vi "Scan_change.vi"() -> ()   [LabVIEW 2022 SP3]
uses:
  <vilib>/userdefined/High Color/IMAQdx.ctl
  <vilib>/vision/driver/IMAQdx.llb/IMAQdx Acquisition Mode.ctl
  <vilib>/vision/driver/IMAQdx.llb/IMAQdx Buffer Number Mode.ctl
  <vilib>/Platform/TimedLoop/XDataNode/timing_clust.ctl
  <vilib>/Platform/TimedLoop/XDataNode/nitl_modes.ctl
  <vilib>/Platform/TimedLoop/XDataNode/wakeup.ctl
  <vilib>/Utility/file.llb/Write To Spreadsheet File (DBL).vi
  <vilib>/Utility/file.llb/Write To Spreadsheet File (I64).vi
  <vilib>/Platform/TimedLoop/XDataNode/XDataNode.xnode
  <vilib>/vision/driver/NI_Vision_Acquisition_Software.lvlib
  <resource>/objmgr/IMAQImage.rc
  <vilib>/Platform/TimedLoop/XDataNode/XDNodeRunTimeDep.lvlib
panel:
  in  "ExitSendCmd":bool
  out "Current File":path
  in  "Root File Name":string="Sample"
  in  "Display as wavelength?":bool=TRUE
  out "X axis":sgl[](array[numeric])
  in  "Tab Control":enum32{"Scan", "Motors"}(tab)
  in  "Release Scan":bool
  in  "Save Option":bool=TRUE
  out "Remaining Minutes":i32
  out "Progress Bar":dbl(slide) scale=0.0..1.0
  in  "Sample #":u16
  out "Cross Plane Length (mm)":sgl=128.0 format="%.3f"
  out "Scan Plane Length (mm)":sgl=128.0 format="%.3f"
  in  "Distance between\nscan lines (mm)":sgl=1.0 min=0.06 max=1000 step=0.06
  in  "Distance between\nplanes (mm)":sgl=1.0 min=0.06 max=1000 step=0.06
  in  "number of planes":u16=1660
  in  "lines per plane":u16=1660 min=1
  out "current plane":u16
  out "current line":u16
  in  "Abort":bool
  in  "start scan":bool
  out "Image":T1(plugin-control)
  out "Spectra":T2(graph)
  in  "Save Folder":path=path "C:/Scan Test"
  in  "Average#":i32=1 min=1
  in  "Exposure (*2.375 ms)":u16=2 format="%.3f"
  in  "Old way (T)/New Way (F)":bool=TRUE
  in  "Plane Axis":refnum<k7>(container)
  in  "Line axis":refnum<k7>(container)
  in  "Home Seq":bool
  in  "Go Home":bool
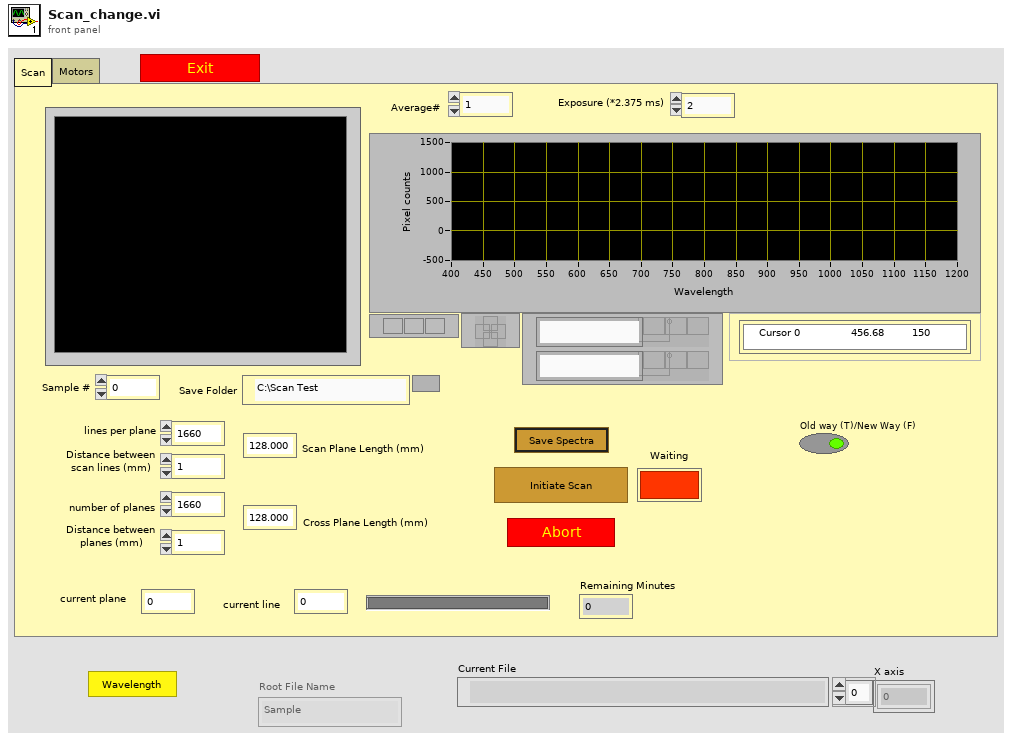
[diagram p1: front panel]
types:
  T1 = typedef "IMAQ Image.ctl" = refnum<image>
  T2 = cluster{"X axis":sgl[], "Spectral Amplitude":dbl[]}
  T3 = typedef "NI_Vision_Acquisition_Software.lvlib/IMAQdx Acquisition Mode.ctl" = enum32{"One Shot", "Continuous"}
  T4 = typedef "IMAQdx.ctl" = refnum<k21>
  T5 = typedef "NI_Vision_Acquisition_Software.lvlib/IMAQdx Buffer Number Mode.ctl" = enum32{"Next", "Last", "Buffer Number", "Every", "Last New"}
  T6 = enum16{"open", "replace", "create", "open or create", "replace or create", "replace or create with confirmation"}
  T7 = typedef "XDNodeRunTimeDep.lvlib/timing_clust.ctl" = cluster{"Expected End [f-1]":u64, "Actual End [f-1]":u64, "Finished Late? [f-1]":bool, "Expected End [i-1]":u64, "Actual End [i-1]":u64, "Finished Late? [i-1]":bool, "Expected Start [i]":u64, "Actual Start [i]":u64, "Expected Start [f]":u64, "Actual Start [f]":u64, "Source Name":string, "Structure Name":string, "Period":i64, "Deadline":i64, "Offset":i64, "Start":i64, "Priority":i32, "Timeout":i32, "Mode":T8, "Wakeup Reason":T9, "Error":errorcluster, "Source Type":string, "Secondary Source Type":string, "Global End Time":u64, "Global Start Time":u64, "Frame Duration":u64, "Iteration Duration":u64, "Assigned CPU":i32, "I/O Scan Engine Mode":u32}
  T8 = typedef "XDNodeRunTimeDep.lvlib/nitl_modes.ctl" = enum32{"No Change", "Process missed periods, maintain original phase", "Discard missed periods, maintain original phase", "Process missed periods, ignore original phase", "Discard missed periods, ignore original phase"}
  T9 = typedef "XDNodeRunTimeDep.lvlib/wakeup.ctl" = enum32{"Normal", "Aborted", "Asynchronous wakeup", "Timing source error", "Timed loop error", "Timeout"}
  T10 = enum16{"big-endian, network order", "native, host order", "little-endian"}
  T11 = typedef "Image Type" = u32
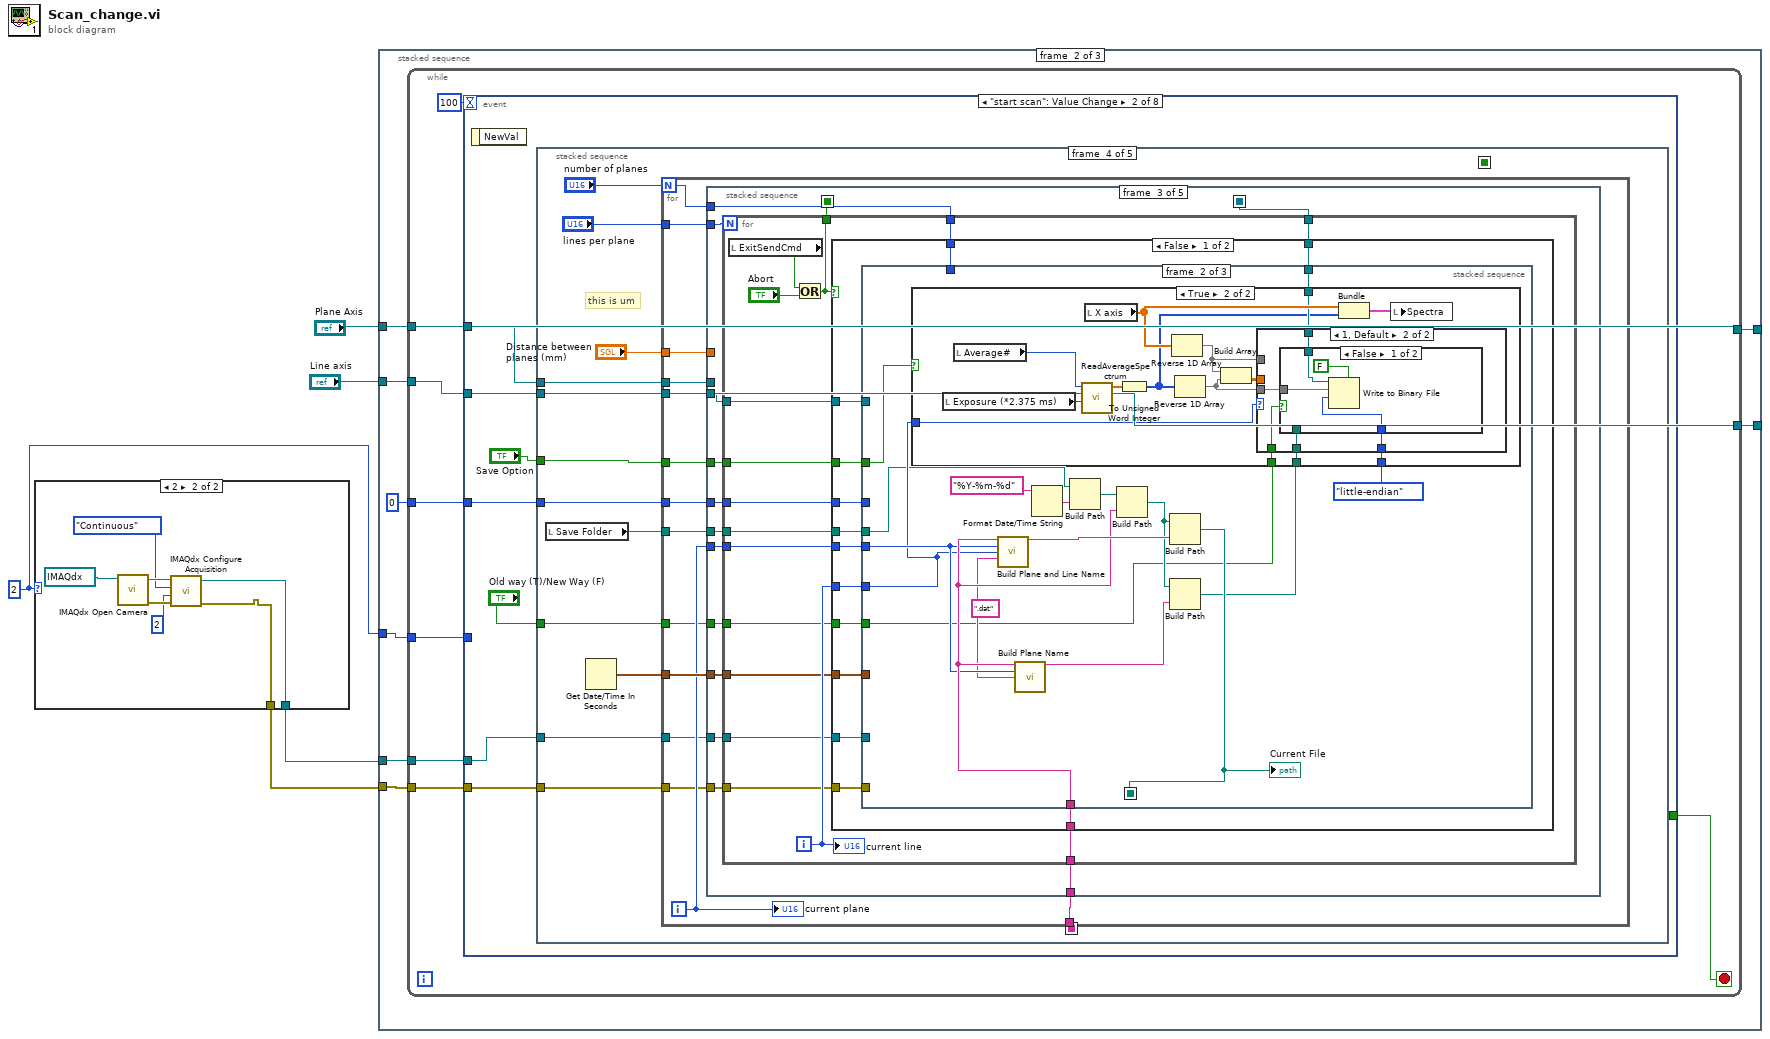
[diagram p0: block diagram]
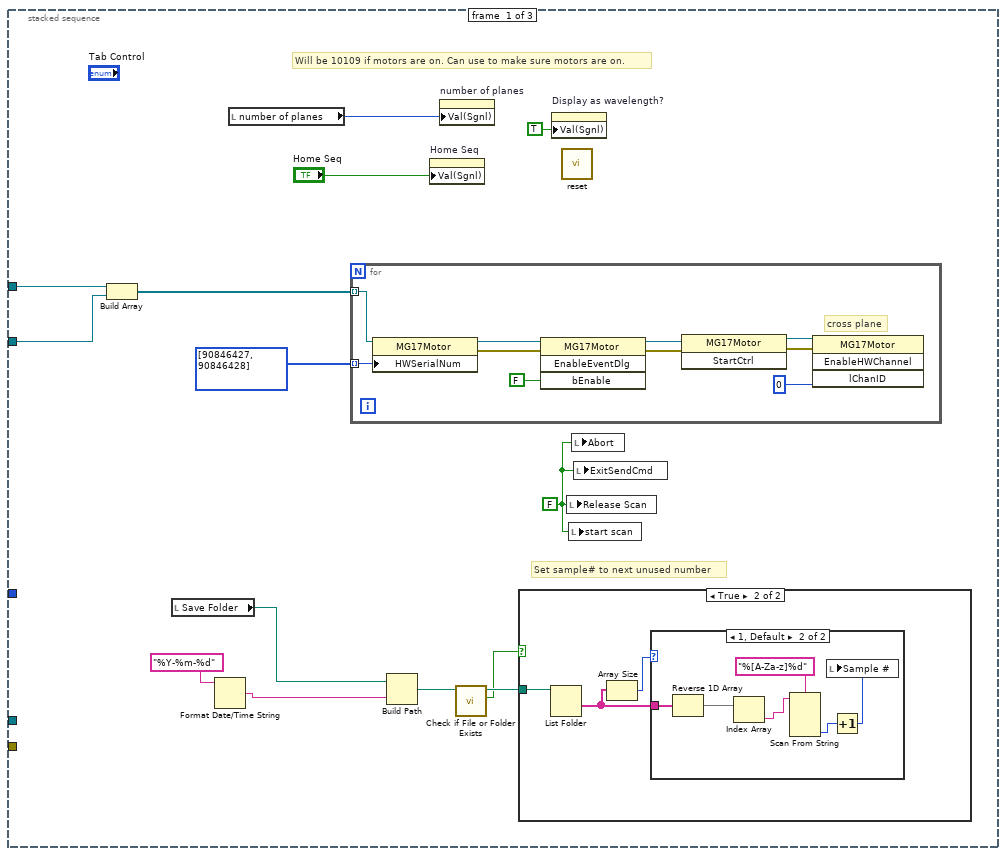
[diagram p3: hidden frame]
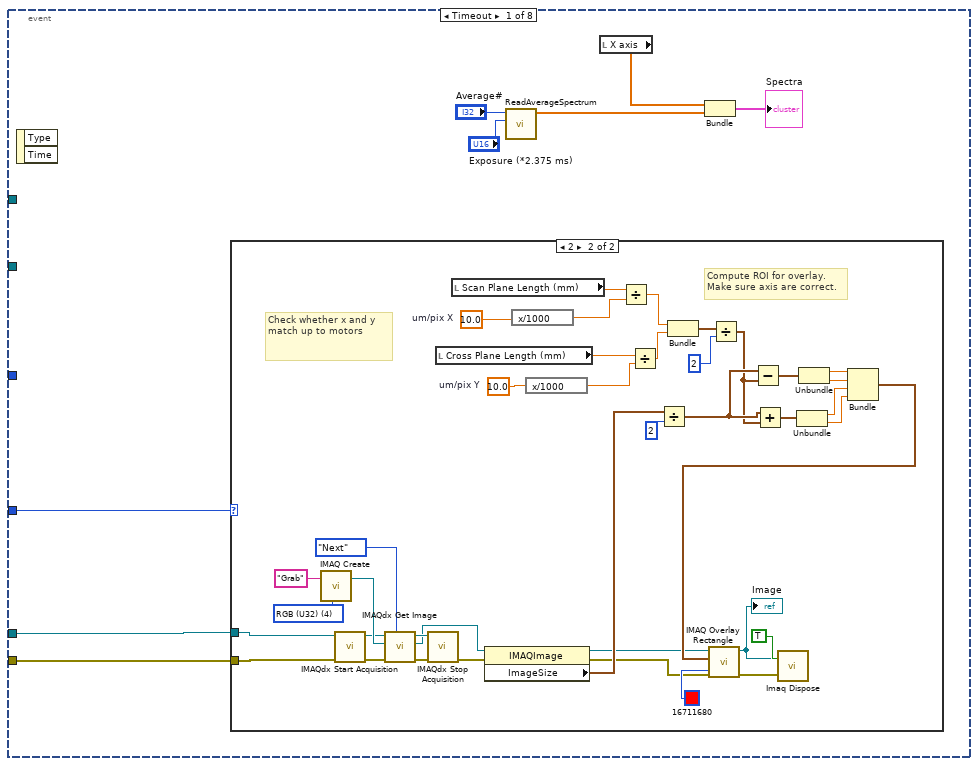
[diagram p6: hidden frame]
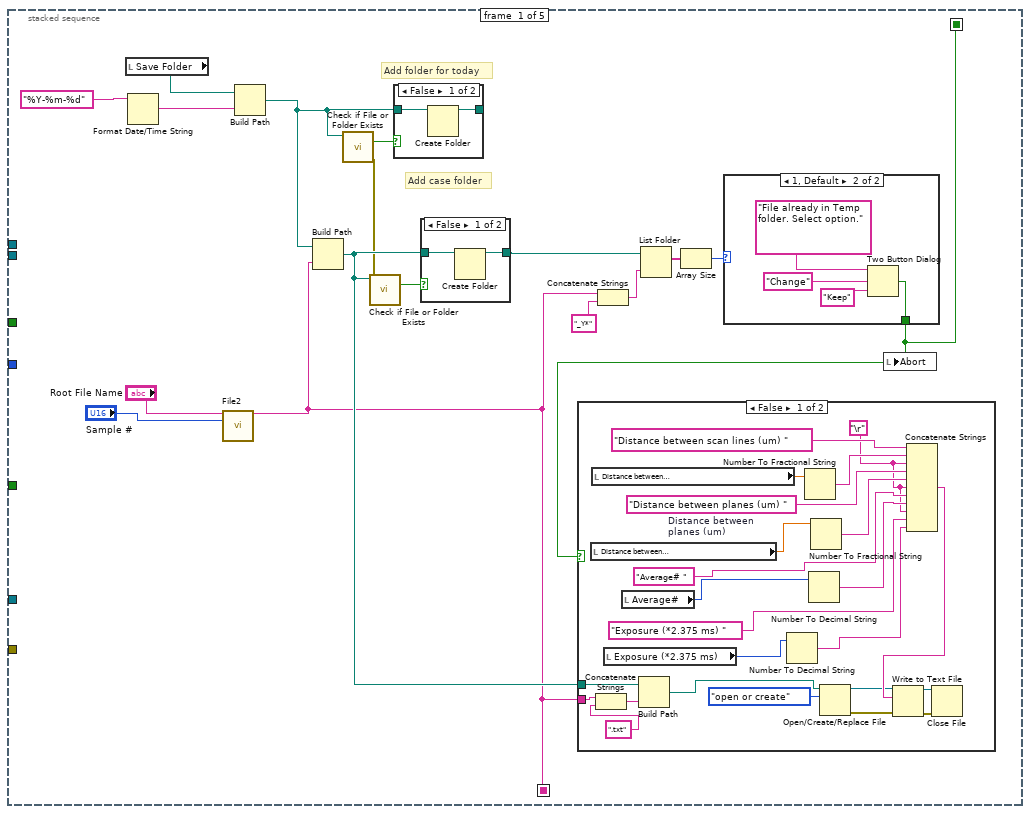
[diagram p8: hidden frame]
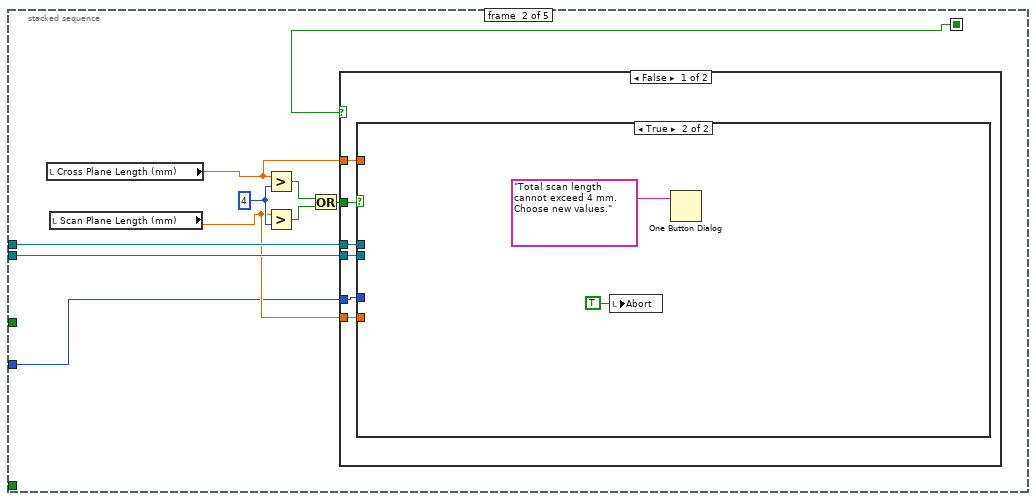
[diagram p13: hidden frame]
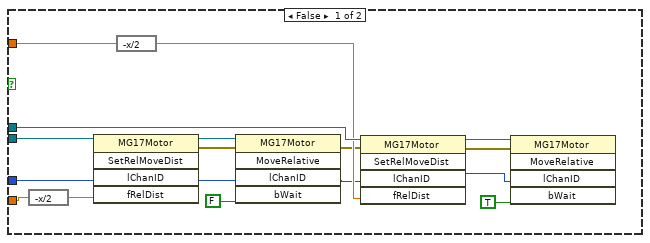
[diagram p14: hidden frame]
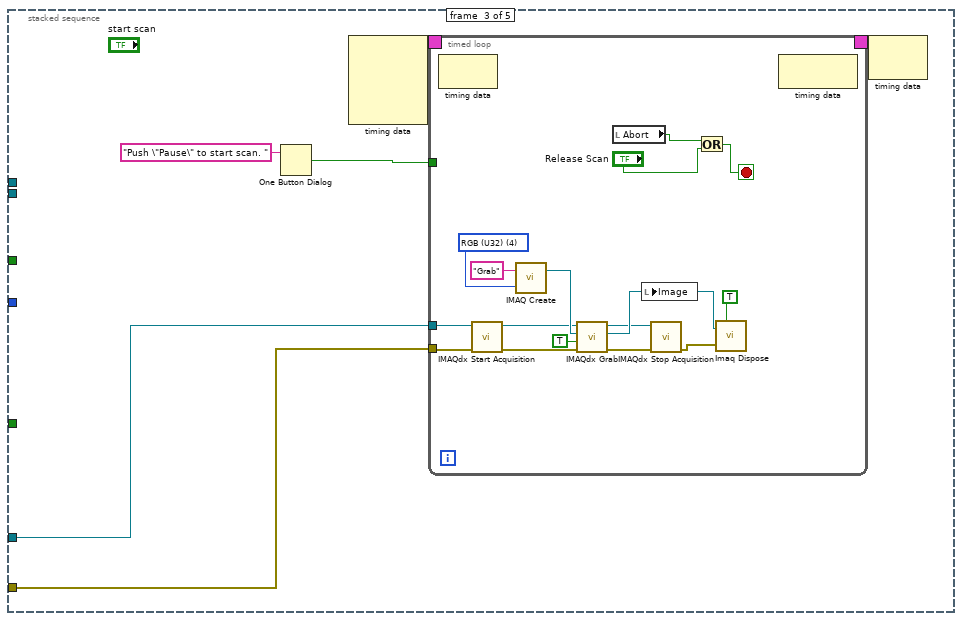
[diagram p16: hidden frame]
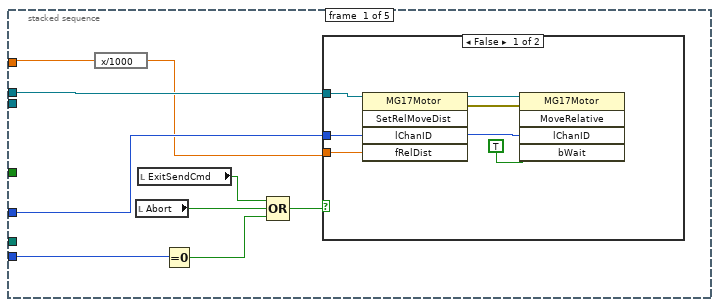
[diagram p17: hidden frame]
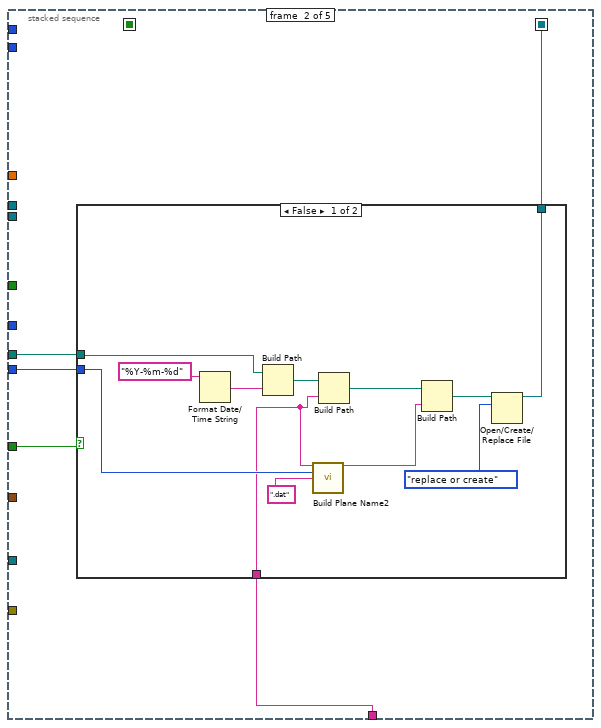
[diagram p19: hidden frame]
diagram:
  w1 = 2 ("bConvert")
  n1 = case shown="2" w1 {
    tunnel: [_ w7] -> w3
    tunnel: [_ w6] -> w2
    frame 0, Default {
    }
    frame 2 {
      n2 = call <vilib>:"IMAQdx Open Camera.vi"("Session In"=T4 "HSC") -> ("error out"=w10:errorcluster, "Session Out"=w11:T4)  [unwired: 2 in, 7 out]
      n3 = call <vilib>:"IMAQdx Configure Acquisition.vi"("error in"=w10, "Number of Buffers"=u32 2, "Continuous?"=IMAQdx_Acquisition_Mode."Continuous", "Session In"=w11) -> ("error out"=w6:errorcluster, "Session Out"=w7:T4)  [unwired: 6 out]
    }
  }
  n4 = stacked-sequence {
    tunnel: [_ w52 _] -> _
    tunnel: [_ w51 _] -> _
    tunnel: "Plane Axis" -> [w20 w50 w576]
    tunnel: "Line axis" -> [w21 w49 w575]
    tunnel: w3 -> [_ w48 w574]
    tunnel: w2 -> [_ w47 w573]
    tunnel: w1 -> [_ w46 w572]
    frame #0 {
      w13 = FALSE ("Release Scan")
      # "Set sample# to next unused number"
      # "Will be 10109 if motors are on. Can use to make sure motors are on."
      n5 = Build Array(w20, w21) -> (w22:refnum<k7>[])
      n6 = local read "Save Folder"() -> (w17:path)
      n7 = Format Date/Time String(time format string (%c)="%Y-%m-%d") -> (date/time string=w18:string)  [unwired: 2 in]
      n8 = local read "number of planes"() -> (w25:u16)
      n9 = for {
        tunnel: i32[] [90846427, 90846428] -> [w37] mode=indexing
        tunnel: w22 -> [w38] mode=indexing
        # "cross plane"
        n10 = property class="MG17Motor"(reference=w38, "HWSerialNum"=w37) -> (reference out=w36:refnum<k7>, error out=w41:errorcluster)  [unwired: 1 in]
        n11 = invoke class="MG17Motor" method="EnableEventDlg"(reference=w36, error in=w41, "bEnable"=FALSE ("pbCommsOK")) -> (reference out=w40:refnum<k7>, error out=w39:errorcluster)  [unwired: 1 in, 2 out]
        n12 = invoke class="MG17Motor" method="StartCtrl"(reference=w40, error in=w39) -> (reference out=w45:refnum<k7>, error out=w44:errorcluster)  [unwired: 1 in, 1 out]
        n13 = invoke class="MG17Motor" method="EnableHWChannel"(reference=w45, error in=w44, "lChanID"=0) -> ()  [unwired: 1 in, 4 out]
      }
      n14 = Build Path(base path=w17, name or relative path=w18) -> (appended path=w16:path)
      n15 = property on="Home Seq" class="Bool (strict)"("Val(Sgnl)"="Home Seq") -> ()  [unwired: 2 in, 2 out]
      n16 = property on="number of planes" class="DigNum (strict)"("Val(Sgnl)"=w25) -> ()  [unwired: 2 in, 2 out]
      n17 = call <vilib>:"Check if File or Folder Exists.vi"("path"=w16) -> ("file or folder exists?"=w14:bool, "dup path"=w15:path)  [unwired: 8 in, 1 out]
      n18 = case shown="True" w14 {
        tunnel: w15 -> [_ w27]
        frame False {
        }
        frame True {
          n19 = List Folder(path=w27) -> (folder names=w29:string[])  [unwired: 2 in, 4 out]
          n20 = Array Size(array=w29) -> (size(s)=w28:i32)
          n21 = case shown="1, Default" w28 {
            tunnel: w29 -> [_ w34]
            frame 0 {
            }
            frame 1, Default {
              n22 = Reverse 1D Array(array=w34) -> (reversed array=w35:string[])
              n23 = Index Array(array=w35) -> (element=w33:string)  [unwired: 1 in]
              n24 = Scan From String(format string="%[A-Za-z]%d", input string=w33) -> (output 2=w32:i32)  [unwired: 5 in, 3 out]
              n25 = Increment(x=w32) -> (x+1=w31:i32)
              n26 = local write "Sample #"(w31) -> ()
            }
          }
        }
      }
      n27 = property on="Display as wavelength?" class="Bool (strict)"("Val(Sgnl)"=TRUE ("Value (Signaling)")) -> ()  [unwired: 2 in, 2 out]
      n28 = call "reset.vi"() -> ()  [unwired: 1 in]
      n29 = local write "Release Scan"(w13) -> ()
      n30 = local write "start scan"(w13) -> ()
      n31 = local write "Abort"(w13) -> ()
      n32 = local write "ExitSendCmd"(w13) -> ()
    }
    frame #1 {
      n33 = while {
        tunnel: w49 -> [w58]
        tunnel: w50 -> [w59]
        tunnel: 0 ("lChanID") -> [w60]
        tunnel: [w58] -> w52
        tunnel: [w59] -> w51
        tunnel: w48 -> [w56]
        tunnel: w47 -> [w55]
        tunnel: w46 -> [w54]
        stop <- w61 stop-if-true
        n34 = event shown="[1] \"start scan\": Value Change" {
          selector: _ -> [_ _ _ _ _ _ _ _]
          dyn-events: _ -> [_ _ _ _ _ _ _ _]
          timeout: 100 -> [_ _ _ _ _ _ _ _]
          tunnel: w58 -> [_ w113 w479 _ w512 _ _ _]
          tunnel: w59 -> [_ w115 w478 _ w513 _ _ _]
          tunnel: [_ _ _ "ExitSendCmd" _ _ _ _] -> w61
          tunnel: w60 -> [_ w114 w474 _ w509 _ _ _]
          tunnel: w56 -> [w64 w112 _ _ _ _ _ _]
          tunnel: w55 -> [w63 w111 _ _ _ _ _ _]
          tunnel: w54 -> [w62 _ _ _ _ _ _ _]
          event Timeout {
            n35 = event-data() -> ()  [unwired: 1 in, 2 out]
            n36 = case shown="2" w62 {
              tunnel: w64 -> [_ w107]
              tunnel: w63 -> [_ w75]
              frame 0, Default {
              }
              frame 2 {
                w81 = T11 4 items=["Grayscale (U8)", "Grayscale (I16)", "Grayscale (SGL)", "Complex (CSG)", "RGB (U32)", "HSL (U32)", "RGB (U64)", "Grayscale (U16)"] ("Image Type")
                w102 = 10.0  # um/pix Y
                w103 = 10.0  # um/pix X
                # "Check whether x and y match up to motors"
                # "Compute ROI for overlay.\nMake sure axis are correct."
                n37 = call "IMAQ Create"("Image Name"="Grab", "Image Type"=w81) -> ("New Image"=w82:T1)  [unwired: 2 in, 2 out]
                n38 = call <vilib>:"IMAQdx Start Acquisition.vi"("error in"=w75, "Session In"=w107) -> ("error out"=w76:errorcluster, "Session Out"=w77:T4)  [unwired: 8 in]
                n39 = call <vilib>:"IMAQdx Get Image.vi"("Buffer Number Mode (Next)"=IMAQdx_Buffer_Number_Mode."Next", "error in"=w76, "Image In"=w82, "Session In"=w77) -> ("error out"=w73:errorcluster, "Image Out"=w71:T1, "Session Out"=w74:T4)  [unwired: 4 in, 1 out]
                n40 = call <vilib>:"IMAQdx Stop Acquisition.vi"("error in"=w73, "Session In"=w74) -> ("error out"=w72:errorcluster)  [unwired: 8 in, 1 out]
                n41 = local read "Cross Plane Length (mm)"() -> (w87:sgl)
                n42 = local read "Scan Plane Length (mm)"() -> (w104:sgl)
                n43 = property class="IMAQImage"(reference=w71, error in=w72) -> (reference out=w70:T1, error out=w79:errorcluster, "ImageSize"=w106:cluster{"x":i32, "y":i32})
                n44 = expression code="x/1000"(w103) -> (w101:dbl)
                n45 = expression code="x/1000"(w102) -> (w86:dbl)
                n46 = Divide(x=w104, y=w101) -> (x/y=w100:dbl)
                n47 = Divide(x=w87, y=w86) -> (x/y=w99:dbl)
                n48 = Divide(x=w106, y=2) -> (x/y=w96:cluster{"x":dbl, "y":dbl})
                n49 = Bundle(w100, w99) -> (w98:cluster{dbl, dbl})  [unwired: 1 in]
                n50 = Divide(x=w98, y=2) -> (x/y=w95:cluster{dbl, dbl})
                n51 = Subtract(x=w96, y=w95) -> (x-y=w94:cluster{dbl, dbl})
                n52 = Add(x=w96, y=w95) -> (x+y=w93:cluster{dbl, dbl})
                n53 = Unbundle(w93) -> (w90:dbl, w89:dbl)
                n54 = Unbundle(w94) -> (w92:dbl, w91:dbl)
                n55 = Bundle(w92, w91, w90, w89) -> (w88:cluster{dbl, dbl, dbl, dbl})  [unwired: 1 in]
                n56 = call "IMAQ Overlay Rectangle"("Color"=u32 16711680, "error in (no error)"=w79, "Rectangle"=w88, "Image"=w70) -> ("error out"=w83:errorcluster, "Image Out"=w84:T1)  [unwired: 6 in]
                "Image" <- w84
                n57 = call "Imaq Dispose"("All Images? (No)"=TRUE, "Image"=w84, "error in (no error)"=w83) -> ()  [unwired: 3 in, 1 out]
              }
            }
            n58 = call "ReadAverageSpectrum.vi"("Exposure (*2.375 ms)"="Exposure (*2.375 ms)", "Average#"="Average#") -> ("Spectral Amplitude"=w65:dbl[])  [unwired: 9 in]
            n59 = local read "X axis"() -> (w69:sgl[])
            n60 = Bundle("X axis"=w69, "Spectral Amplitude"=w65) -> (→"Spectra":T2)  [unwired: 1 in]
          }
          event "start scan": Value Change {
            n61 = event-data() -> ()  [unwired: 1 in, 1 out]
            n62 = stacked-sequence {
              seq-local: [w120 _ _ _ _] -> [_ _ _ w236 _]
              seq-local: [w116 _ _ _ _] -> [_ w167 _ _ _]
              tunnel: w115 -> [_ w172 _ w240 _]
              tunnel: w113 -> [_ w173 _ w238 _]
              tunnel: w114 -> [_ w168 _ w237 _]
              tunnel: w112 -> [_ _ w207 w232 _]
              tunnel: w111 -> [_ _ w206 w231 _]
              tunnel: "Save Option" -> [_ _ _ w230 _]
              tunnel: "Old way (T)/New Way (F)" -> [_ _ _ w228 _]
              frame #0 {
                # "Add folder for today"
                # "Add case folder"
                n63 = local read "Save Folder"() -> (w127:path)
                n64 = Format Date/Time String(time format string (%c)="%Y-%m-%d") -> (date/time string=w128:string)  [unwired: 2 in]
                n65 = call "File2"("Beginning Text"="Root File Name", "d"="Sample #") -> ("Result"=w120:string)  [unwired: 12 in, 1 out]
                n66 = Build Path(base path=w127, name or relative path=w128) -> (appended path=w118:path)
                n67 = Build Path(base path=w118, name or relative path=w120) -> (appended path=w121:path)
                n68 = call <vilib>:"Check if File or Folder Exists.vi"("path"=w118) -> ("error out"=w117:errorcluster, "file or folder exists?"=w119:bool)  [unwired: 8 in, 1 out]
                n69 = call <vilib>:"Check if File or Folder Exists.vi"("error in (no error)"=w117, "path"=w121) -> ("file or folder exists?"=w124:bool)  [unwired: 7 in, 2 out]
                n70 = case shown="False" w119 {
                  tunnel: w118 -> [w134 w135]
                  tunnel: [w133 w135] -> _
                  frame False {
                    n71 = Create Folder(path (use dialog)=w134) -> (created path=w133:path)  [unwired: 2 in, 2 out]
                  }
                  frame True {
                  }
                }
                n72 = case shown="False" w124 {
                  tunnel: w121 -> [w165 w166]
                  tunnel: [w164 w166] -> w122
                  frame False {
                    n73 = Create Folder(path (use dialog)=w165) -> (created path=w164:path)  [unwired: 2 in, 2 out]
                  }
                  frame True {
                  }
                }
                n74 = Concatenate Strings(w120, "_Y*") -> (w132:string)
                n75 = List Folder(path=w122, pattern=w132) -> (filenames=w131:string[])  [unwired: 1 in, 4 out]
                n76 = Array Size(array=w131) -> (size(s)=w130:i32)
                n77 = case shown="1, Default" w130 {
                  tunnel: [_ w160] -> w116
                  frame 0 {
                  }
                  frame 1, Default {
                    n78 = Two Button Dialog(message="File already in Temp folder. Select option.", 1:"Keep" ("F button name (\"Cancel\")"), 2:"Change" ("T button name (\"OK\")")) -> (T button?=w160:bool)
                  }
                }
                n79 = case shown="False" w116 {
                  tunnel: w121 -> [w147 _]
                  tunnel: w120 -> [w146 _]
                  frame False {
                    w136 = "\r"
                    w150 = "Distance between planes (um) "  # Distance between planes (um)
                    n80 = local read "Distance between\nplanes (mm)"() -> (w158:sgl)
                    n81 = local read "Distance between\nscan lines (mm)"() -> (w159:sgl)
                    n82 = Concatenate Strings(w146, ".txt") -> (w145:string)
                    n83 = local read "Exposure (*2.375 ms)"() -> (w156:u16)
                    n84 = local read "Average#"() -> (w157:i32)
                    n85 = Build Path(base path=w147, name or relative path=w145) -> (appended path=w141:path)
                    n86 = Number To Decimal String(number=w156) -> (decimal integer string=w148:string)  [unwired: 1 in]
                    n87 = Number To Fractional String(number=w159) -> (F-format string=w154:string)  [unwired: 3 in]
                    n88 = Number To Decimal String(number=w157) -> (decimal integer string=w151:string)  [unwired: 1 in]
                    n89 = Number To Fractional String(number=w158) -> (F-format string=w153:string)  [unwired: 3 in]
                    n90 = Open/Create/Replace File(file path (use dialog)=w141, operation (0:open)=T6."open or create") -> (refnum out=w140:refnum<file>, error out=w139:errorcluster)  [unwired: 4 in, 1 out]
                    n91 = Concatenate Strings("Distance between scan lines (um) ", w154, w136, w150, w153, w136, "Average# ", w151, w136, "Exposure (*2.375 ms) ", w148) -> (w143:string)
                    n92 = Write to Text File(file (use dialog)=w140, text=w143, error in=w139) -> (refnum out=w137:refnum<file>, error out=w138:errorcluster)  [unwired: 1 in, 1 out]
                    n93 = Close File(refnum=w137, error in=w138) -> ()  [unwired: 2 out]
                  }
                  frame True {
                  }
                }
                n94 = local write "Abort"(w116) -> ()
              }
              frame #1 {
                w175 = 4
                n95 = local read "Cross Plane Length (mm)"() -> (w171:sgl)
                n96 = local read "Scan Plane Length (mm)"() -> (w170:sgl)
                n97 = Greater?(x=w171, y=w175) -> (0:w176:bool)
                n98 = Greater?(x=w170, y=w175) -> (0:w174:bool)
                n99 = Or(x=w176, y=w174) -> (x .or. y?=w169:bool)
                n100 = case shown="False" w167 {
                  tunnel: w173 -> [w182 _]
                  tunnel: w172 -> [w181 _]
                  tunnel: w171 -> [w180 _]
                  tunnel: w170 -> [w179 _]
                  tunnel: w169 -> [w178 _]
                  tunnel: w168 -> [w177 _]
                  frame False {
                    n101 = case shown="True" w178 {
                      tunnel: w182 -> [w193 _]
                      tunnel: w181 -> [w192 _]
                      tunnel: w177 -> [w187 _]
                      tunnel: w180 -> [w191 _]
                      tunnel: w179 -> [w190 _]
                      frame False {
                        n102 = expression code="-x/2"(w190) -> (w189:sgl)
                        n103 = invoke class="MG17Motor" method="SetRelMoveDist"(reference=w193, "lChanID"=w187, "fRelDist"=w189) -> (reference out=w198:refnum<k7>, error out=w184:errorcluster, "lChanID"=w197:i32)  [unwired: 2 in, 2 out]
                        n104 = expression code="-x/2"(w191) -> (w188:sgl)
                        n105 = invoke class="MG17Motor" method="MoveRelative"(reference=w198, error in=w184, "lChanID"=w197, "bWait"=FALSE) -> (error out=w185:errorcluster, "lChanID"=w183:i32)  [unwired: 1 in, 3 out]
                        n106 = invoke class="MG17Motor" method="SetRelMoveDist"(reference=w192, error in=w185, "lChanID"=w183, "fRelDist"=w188) -> (reference out=w195:refnum<k7>, error out=w186:errorcluster, "lChanID"=w194:i32)  [unwired: 1 in, 2 out]
                        n107 = invoke class="MG17Motor" method="MoveRelative"(reference=w195, error in=w186, "lChanID"=w194, "bWait"=TRUE) -> ()  [unwired: 1 in, 5 out]
                      }
                      frame True {
                        n108 = local write "Abort"(TRUE ("Abort")) -> ()
                        n109 = One Button Dialog(message="Total scan length cannot exceed 4 mm. Choose new values.") -> ()  [unwired: 1 in, 1 out]
                      }
                    }
                  }
                  frame True {
                  }
                }
              }
              frame #2 {
                n110 = One Button Dialog(message="Push \"Pause\" to start scan. ") -> (true=w204:bool)  [unwired: 1 in]
                n111 = node-c288() -> (w203:T7)  [unwired: 4 in]
                n112 = timed-loop {
                  tunnel: w207 -> [w217]
                  tunnel: w206 -> [w215]
                  tunnel: w204 -> [_]
                  timing: w203 -> [_]
                  timing-out: [_] -> w202
                  stop <- w209 stop-if-true
                  w218 = T11 4 items=["Grayscale (U8)", "Grayscale (I16)", "Grayscale (SGL)", "Complex (CSG)", "RGB (U32)", "HSL (U32)", "RGB (U64)", "Grayscale (U16)"] ("Image Type")
                  n113 = node-c288() -> ()  [unwired: 1 in, 1 out]
                  n114 = call <vilib>:"IMAQdx Start Acquisition.vi"("error in"=w215, "Session In"=w217) -> ("error out"=w216:errorcluster, "Session Out"=w212:T4)  [unwired: 8 in]
                  n115 = call "IMAQ Create"("Image Name"="Grab", "Image Type"=w218) -> ("New Image"=w219:T1)  [unwired: 2 in, 2 out]
                  n116 = call <vilib>:"IMAQdx Grab.vi"("error in"=w216, "Wait for Next Buffer? (Yes)"=TRUE, "Image In"=w219, "Session In"=w212) -> ("error out"=w214:errorcluster, "Image Out"=w221:T1, "Session Out"=w211:T4)  [unwired: 5 out]
                  n117 = local read "Abort"() -> (w208:bool)
                  n118 = local write "Image"(w221) -> ()
                  n119 = call <vilib>:"IMAQdx Stop Acquisition.vi"("error in"=w214, "Session In"=w211) -> ("error out"=w213:errorcluster)  [unwired: 8 in, 1 out]
                  n120 = Or(x=w208, y="Release Scan") -> (x .or. y?=w209:bool)
                  n121 = call "Imaq Dispose"("All Images? (No)"=TRUE, "Image"=w221, "error in (no error)"=w213) -> ()  [unwired: 3 in, 1 out]
                  n122 = node-c288() -> ()  [unwired: 1 in, 1 out]
                }
                n123 = node-c288(w202) -> ()  [unwired: 1 out]
              }
              frame #3 {
                # "this is um"
                n124 = local read "Save Folder"() -> (w229:path)
                n125 = Get Date/Time In Seconds() -> (seconds since 1Jan1904=w233:timestamp)
                n126 = for {
                  N: "number of planes" -> [w243]
                  tunnel: "lines per plane" -> [w254]
                  tunnel: w240 -> [w253]
                  tunnel: "Distance between\nplanes (mm)" -> [w252]
                  tunnel: w238 -> [w251]
                  tunnel: w237 -> [w250]
                  tunnel: w236 -> [w249]
                  tunnel: w233 -> [w248]
                  tunnel: w232 -> [w246]
                  tunnel: w231 -> [w245]
                  tunnel: w230 -> [w244]
                  tunnel: w229 -> [w242]
                  tunnel: w228 -> [w241]
                  i -> [w247]
                  n127 = stacked-sequence {
                    seq-local: [_ _ w293 _ _] -> [_ _ _ w440 _]
                    seq-local: [_ w271 _ _ _] -> [_ _ w288 w438 _]
                    tunnel: w254 -> [_ _ w291 _ _]
                    tunnel: w253 -> [w263 _ _ _ _]
                    tunnel: w252 -> [w261 _ _ _ _]
                    tunnel: w251 -> [_ _ w292 w441 _]
                    tunnel: w250 -> [w262 _ w301 w442 _]
                    tunnel: w247 -> [w256 w275 w300 _ w454]
                    tunnel: w249 -> [_ w273 w299 _ _]
                    tunnel: w243 -> [_ _ w298 _ w455]
                    tunnel: w248 -> [_ _ w297 _ w456]
                    tunnel: w246 -> [_ _ w296 _ _]
                    tunnel: w245 -> [_ _ w295 _ _]
                    tunnel: w244 -> [_ _ w294 _ _]
                    tunnel: w242 -> [_ w274 w290 _ _]
                    tunnel: w241 -> [_ w272 w289 w439 _]
                    frame #0 {
                      n128 = expression code="x/1000"(w261) -> (w260:sgl)
                      n129 = local read "Abort"() -> (w259:bool)
                      n130 = local read "ExitSendCmd"() -> (w255:bool)
                      n131 = Equal To 0?(x=w256) -> (x = 0?=w258:bool)
                      n132 = Compound Arithmetic op=OR(w255, w259, w258) -> (w257:bool)
                      n133 = case shown="False" w257 {
                        tunnel: w263 -> [w269 _]
                        tunnel: w262 -> [w266 _]
                        tunnel: w260 -> [w265 _]
                        frame False {
                          n134 = invoke class="MG17Motor" method="SetRelMoveDist"(reference=w269, "lChanID"=w266, "fRelDist"=w265) -> (reference out=w268:refnum<k7>, error out=w264:errorcluster, "lChanID"=w267:i32)  [unwired: 2 in, 2 out]
                          n135 = invoke class="MG17Motor" method="MoveRelative"(reference=w268, error in=w264, "lChanID"=w267, "bWait"=TRUE) -> ()  [unwired: 1 in, 5 out]
                        }
                        frame True {
                        }
                      }
                    }
                    frame #1 {
                      n136 = case shown="False" w272 {
                        tunnel: w275 -> [w285 _]
                        tunnel: w274 -> [w281 _]
                        tunnel: w273 -> [w280 _]
                        tunnel: [w276 _] -> w271
                        frame False {
                          n137 = Format Date/Time String(time format string (%c)="%Y-%m-%d") -> (date/time string=w284:string)  [unwired: 2 in]
                          n138 = Build Path(base path=w281, name or relative path=w284) -> (appended path=w282:path)
                          n139 = call "Build Plane Name2"("Beginning Text"=w280, "plane"=w285, "file_EXT"=".dat") -> ("Result"=w286:string)  [unwired: 11 in, 1 out]
                          n140 = Build Path(base path=w282, name or relative path=w280) -> (appended path=w279:path)
                          n141 = Build Path(base path=w279, name or relative path=w286) -> (appended path=w278:path)
                          n142 = Open/Create/Replace File(file path (use dialog)=w278, operation (0:open)=T6."replace or create") -> (refnum out=w276:refnum<file>)  [unwired: 4 in, 2 out]
                        }
                        frame True {
                        }
                      }
                    }
                    frame #2 {
                      n143 = for {
                        N: w291 -> [_]
                        tunnel: w292 -> [w317]
                        tunnel: w301 -> [w316]
                        tunnel: w300 -> [w314]
                        tunnel: w299 -> [w313]
                        tunnel: w298 -> [w312]
                        tunnel: w297 -> [w311]
                        tunnel: w296 -> [w310]
                        tunnel: w295 -> [w309]
                        tunnel: w294 -> [w308]
                        tunnel: [w305] -> w293
                        tunnel: w290 -> [w304]
                        tunnel: w289 -> [w303]
                        tunnel: w288 -> [w302]
                        i -> [w315]
                        n144 = local read "ExitSendCmd"() -> (w307:bool)
                        n145 = Or(x=w307, y="Abort") -> (x .or. y?=w305:bool)
                        n146 = case shown="False" w305 {
                          tunnel: w317 -> [w330 _]
                          tunnel: w316 -> [w329 _]
                          tunnel: w315 -> [w328 _]
                          tunnel: w314 -> [w327 _]
                          tunnel: w313 -> [w326 _]
                          tunnel: w312 -> [w325 _]
                          tunnel: w311 -> [w324 _]
                          tunnel: w310 -> [w323 _]
                          tunnel: w309 -> [w322 _]
                          tunnel: w308 -> [w321 _]
                          tunnel: w304 -> [w320 _]
                          tunnel: w303 -> [w319 _]
                          tunnel: w302 -> [w318 _]
                          frame False {
                            n147 = stacked-sequence {
                              seq-local: [_ w360 _] -> [_ _ w413]
                              tunnel: w330 -> [w333 _ _]
                              tunnel: w329 -> [w332 _ _]
                              tunnel: w328 -> [w331 w349 _]
                              tunnel: w327 -> [_ w353 _]
                              tunnel: w326 -> [_ w354 _]
                              tunnel: w325 -> [_ _ _]
                              tunnel: w324 -> [_ _ _]
                              tunnel: w323 -> [_ _ w414]
                              tunnel: w322 -> [_ _ w411]
                              tunnel: w321 -> [_ w356 w412]
                              tunnel: w320 -> [_ w347 _]
                              tunnel: w319 -> [_ w346 _]
                              tunnel: w318 -> [_ w345 _]
                              frame #0 {
                                n148 = case shown="1, Default" w331 {
                                tunnel: w333 -> [_ w341]
                                tunnel: w332 -> [_ w340]
                                tunnel: [_ w336] -> _
                                tunnel: [_ w335] -> _
                                frame 0 {
                                }
                                frame 1, Default {
                                # "this is um"
                                n149 = expression code="x/1000"("Distance between\nscan lines (mm)") -> (w338:sgl)
                                n150 = invoke class="MG17Motor" method="SetRelMoveDist"(reference=w341, "lChanID"=w340, "fRelDist"=w338) -> (reference out=w343:refnum<k7>, error out=w339:errorcluster, "lChanID"=w342:i32)  [unwired: 2 in, 2 out]
                                n151 = invoke class="MG17Motor" method="MoveRelative"(reference=w343, error in=w339, "lChanID"=w342, "bWait"=TRUE) -> (error out=w336:errorcluster, "bWait"=w335:bool)  [unwired: 1 in, 3 out]
                                }
                                }
                              }
                              frame #1 {
                                w352 = ".dat" ("file_EXT")
                                n152 = call "Build Plane and Line Name"("Beginning Text"=w354, "plane"=w353, "line"=w349, "file_EXT"=w352) -> ("Result"=w359:string)  [unwired: 10 in, 1 out]
                                n153 = call "Build Plane Name"("Beginning Text"=w354, "plane"=w353, "file_EXT"=w352) -> ("Result"=w351:string)  [unwired: 11 in, 1 out]
                                n154 = Format Date/Time String(time format string (%c)="%Y-%m-%d") -> (date/time string=w358:string)  [unwired: 2 in]
                                n155 = Build Path(base path=w347, name or relative path=w358) -> (appended path=w355:path)
                                n156 = Build Path(base path=w355, name or relative path=w354) -> (appended path=w350:path)
                                n157 = Build Path(base path=w350, name or relative path=w359) -> (appended path=w360:path)
                                "Current File" <- w360
                                n158 = Build Path(base path=w350, name or relative path=w351) -> (appended path=w344:path)
                                n159 = case shown="True" w356 {
                                tunnel: w349 -> [_ w369]
                                tunnel: w346 -> [_ w367]
                                tunnel: w344 -> [_ w365]
                                tunnel: T10."little-endian" ("byte order (0:big-endian, network order)") -> [_ w364]
                                tunnel: w345 -> [_ w363]
                                frame False {
                                }
                                frame True {
                                n160 = local read "Exposure (*2.375 ms)"() -> (w372:u16)
                                n161 = local read "Average#"() -> (w373:i32)
                                n162 = call "ReadAverageSpectrum.vi"("Exposure (*2.375 ms)"=w372, "Average#"=w373) -> ("Spectral Amplitude"=w366:dbl[])  [unwired: 9 in]
                                n163 = local read "X axis"() -> (w371:sgl[])
                                n164 = To Unsigned Word Integer(number=w366) -> (unsigned 16bit integer=w362:u16[])
                                n165 = Reverse 1D Array(array=w371) -> (reversed array=w361:sgl[])
                                n166 = Reverse 1D Array(array=w362) -> (reversed array=w368:u16[])
                                n167 = Build Array(w361, w368) -> (w374:sgl[][])
                                n168 = case shown="1, Default" w369 {
                                tunnel: w374 -> [w381 _]
                                tunnel: w368 -> [w375 w401]
                                tunnel: w367 -> [w380 w400]
                                tunnel: w365 -> [w379 w398]
                                tunnel: w364 -> [w378 w399]
                                tunnel: w363 -> [w377 w397]
                                tunnel: w361 -> [w376 _]
                                frame 0 {
                                n169 = case shown="False" w380 {
                                tunnel: w381 -> [_ w396]
                                tunnel: w379 -> [_ w393]
                                tunnel: w378 -> [w385 _]
                                tunnel: w377 -> [w391 _]
                                tunnel: w376 -> [w384 _]
                                tunnel: w375 -> [w383 _]
                                frame False {
                                w386 = FALSE ("prepend array or string size? (T)")
                                n170 = Array Size(array=w384) -> (size(s)=w392:i32)
                                n171 = To Word Integer(number=w392) -> (16bit integer=w382:i16)
                                n172 = Write to Binary File(file (use dialog)=w391, data=w382, 5:w386, 9:w385) -> (refnum out=w387:refnum<file>, error out=w390:errorcluster)  [unwired: 2 in, 1 out]
                                n173 = Write to Binary File(file (use dialog)=w387, data=w384, error in=w390, 5:w386, 9:w385) -> (refnum out=w388:refnum<file>, error out=w389:errorcluster)  [unwired: 1 in, 1 out]
                                n174 = Write to Binary File(file (use dialog)=w388, data=w383, error in=w389, 5:w386, 9:w385) -> ()  [unwired: 1 in, 3 out]
                                }
                                frame True {
                                n175 = call-poly <vilib>:"Write To Spreadsheet File.vi"("delimiter (\\t)"="\t" ("delimiter (\\t)"), "transpose? (no:F)"=FALSE, "2D data"=w396, "file path (dialog if empty)"=w393) -> ()  [unwired: 4 in, 1 out]
                                }
                                }
                                }
                                frame 1, Default {
                                n176 = case shown="False" w400 {
                                tunnel: w401 -> [w405 w409]
                                tunnel: w399 -> [w404 _]
                                tunnel: w398 -> [_ w406]
                                tunnel: w397 -> [w402 _]
                                frame False {
                                n177 = Write to Binary File(file (use dialog)=w402, data=w405, 5:FALSE ("prepend array or string size? (T)"), 9:w404) -> ()  [unwired: 2 in, 3 out]
                                }
                                frame True {
                                n178 = call-poly <vilib>:"Write To Spreadsheet File.vi"("delimiter (\\t)"="\t" ("delimiter (\\t)"), "transpose? (no:F)"=FALSE, "append to file? (new file:F)"=TRUE, "1D data"=w409, "file path (dialog if empty)"=w406) -> ()  [unwired: 3 in, 1 out]
                                }
                                }
                                }
                                }
                                n179 = Bundle("X axis"=w371, w362) -> (w370:cluster{"X axis":sgl[], u16[]})  [unwired: 1 in]
                                n180 = local write "Spectra"(w370) -> ()
                                }
                                }
                              }
                              frame #2 {
                                n181 = case shown="False" w412 {
                                tunnel: w414 -> [w420 _]
                                tunnel: w413 -> [w436 _]
                                tunnel: w411 -> [w418 _]
                                frame False {
                                w427 = T11 4 items=["Grayscale (U8)", "Grayscale (I16)", "Grayscale (SGL)", "Complex (CSG)", "RGB (U32)", "HSL (U32)", "RGB (U64)", "Grayscale (U16)"] ("Image Type")
                                n182 = call <vilib>:"IMAQdx Start Acquisition.vi"("error in"=w418, "Session In"=w420) -> ("error out"=w417:errorcluster, "Session Out"=w419:T4)  [unwired: 8 in]
                                n183 = Strip Path(path=w436) -> (stripped path=w416:path, name=w435:string)
                                n184 = call "IMAQ Create"("Image Name"="Grab", "Image Type"=w427, "error in (no error)"=w417) -> ("New Image"=w425:T1, "error out"=w426:errorcluster)  [unwired: 1 in, 1 out]
                                n185 = call <vilib>:"IMAQdx Get Image.vi"("Buffer Number Mode (Next)"=IMAQdx_Buffer_Number_Mode."Next", "error in"=w426, "Image In"=w425, "Session In"=w419) -> ("error out"=w423:errorcluster, "Image Out"=w437:T1, "Session Out"=w421:T4)  [unwired: 4 in, 1 out]
                                n186 = Search and Replace String(input string=w435, search string=".dat", replace string=".jpg" ("search string")) -> (result string=w433:string)  [unwired: 5 in, 3 out]
                                n187 = local write "Image"(w437) -> ()
                                n188 = call <vilib>:"IMAQdx Stop Acquisition.vi"("error in"=w423, "Session In"=w421) -> ("error out"=w422:errorcluster)  [unwired: 8 in, 1 out]
                                n189 = Build Path(base path=w416, name or relative path=w433) -> (appended path=w415:path)
                                n190 = call-poly "IMAQ Write File 2"("error in (no error)"=w422, "File Path"=w415, "Image"=w437) -> ("error out"=w430:errorcluster, "Image Out (duplicate)"=w431:T1)  [unwired: 7 in]
                                n191 = local write "Current File"(w415) -> ()
                                n192 = call "Imaq Dispose"("All Images? (No)"=TRUE, "Image"=w431, "error in (no error)"=w430) -> ()  [unwired: 3 in, 1 out]
                                }
                                frame True {
                                }
                                }
                              }
                            }
                          }
                          frame True {
                          }
                        }
                        "current line" <- w315
                      }
                    }
                    frame #3 {
                      n193 = case shown="False" w440 {
                        tunnel: w442 -> [w446 _]
                        tunnel: w441 -> [w444 _]
                        frame False {
                          n194 = local read "Scan Plane Length (mm)"() -> (w447:sgl)
                          n195 = Negate(x=w447) -> (-x=w445:sgl)
                          n196 = invoke class="MG17Motor" method="SetRelMoveDist"(reference=w444, "lChanID"=w446, "fRelDist"=w445) -> (reference out=w449:refnum<k7>, error out=w451:errorcluster, "lChanID"=w450:i32)  [unwired: 2 in, 2 out]
                          n197 = invoke class="MG17Motor" method="MoveRelative"(reference=w449, error in=w451, "lChanID"=w450, "bWait"=TRUE) -> ()  [unwired: 1 in, 5 out]
                        }
                        frame True {
                        }
                      }
                      n198 = case shown="False" w439 {
                        tunnel: w438 -> [w443 _]
                        frame False {
                          n199 = Close File(refnum=w443) -> ()  [unwired: 1 in, 2 out]
                        }
                        frame True {
                        }
                      }
                    }
                    frame #4 {
                      n200 = Get Date/Time In Seconds() -> (seconds since 1Jan1904=w461:timestamp)
                      n201 = Subtract(x=w461, y=w456) -> (x-y=w460:dbl)
                      n202 = Divide(x=w454, y=w455) -> (x/y=w452:dbl)
                      "Progress Bar" <- w452
                      n203 = Divide(x=w460, y=60) -> (x/y=w457:dbl)
                      n204 = Divide(x=w457, y=w452) -> (x/y=w458:dbl)
                      n205 = Subtract(x=w458, y=w457) -> (x-y=→"Remaining Minutes":dbl)
                    }
                  }
                  "current plane" <- w247
                }
              }
              frame #4 {
                w462 = FALSE ("Start Delay")
                n206 = local read "Abort"() -> (w465:bool)
                n207 = case shown="True" w465 {
                  frame False {
                    n208 = local read "Sample #"() -> (w467:u16)
                    n209 = Increment(x=w467) -> (x+1=w468:u16)
                    n210 = local write "Sample #"(w468) -> ()
                  }
                  frame True {
                    n211 = local write "Abort"(FALSE ("Abort")) -> ()
                  }
                }
                n212 = local write "Remaining Minutes"(0 ("Remaining Minutes")) -> ()
                n213 = local write "Progress Bar"(0.0 ("Progress Bar")) -> ()
                n214 = local write "Release Scan"(w462) -> ()
                n215 = local write "start scan"(w462) -> ()
                n216 = property on="Go Home" class="Bool (strict)"("Val(Sgnl)"="Go Home") -> ()  [unwired: 2 in, 2 out]
              }
            }
          }
          event "Home Seq": Value Change {
            n217 = event-data() -> ()  [unwired: 1 in, 5 out]
            n218 = invoke class="MG17Motor" method="GetStatusBits_Bits"(reference=w478, "lChanID"=w474) -> ("GetStatusBits_Bits"=w477:i32)  [unwired: 2 in, 3 out]
            n219 = Number To Boolean Array(number=w477) -> (Boolean array=w476:bool[])
            n220 = Index Array(array=w476, index=10) -> (element=w472:bool)
            n221 = case shown="True" w472 {
              tunnel: [_ w481] -> w471
              frame False {
              }
              frame True {
                n222 = Two Button Dialog(message="Home Sequence Was Already Performed", 1:"Override" ("F button name (\"Cancel\")")) -> (T button?=w481:bool)  [unwired: 1 in]
              }
            }
            n223 = local write "Home Seq"(FALSE ("Home Seq")) -> ()
            n224 = case shown="False" w471 {
              tunnel: w479 -> [w485 w498]
              tunnel: w474 -> [w487 _]
              tunnel: w478 -> [w486 w499]
              frame False {
                n225 = Build Array(w486, w485) -> (w484:refnum<k7>[])
                n226 = for {
                  tunnel: w487 -> [w497]
                  tunnel: w484 -> [w496] mode=indexing
                  tunnel: bool[] [FALSE, TRUE] -> [w495] mode=indexing
                  w493 = sgl 0.5  # pfPitch
                  w490 = 1  # plDirSense
                  w494 = 1  # plUnits
                  n227 = invoke class="MG17Motor" method="MoveHome"(reference=w496, "lChanID"=w497, "bWait"=w495) -> (reference out=w488:refnum<k7>)  [unwired: 2 in, 4 out]
                  n228 = invoke class="MG17Motor" method="SetStageAxisInfo"(reference=w488, "lChanID"=0 ("lLimitMode"), "fMinPos"=sgl 0.0, "fMaxPos"=sgl 4.0, "lUnits"=w494, "fPitch"=w493, "lDirSense"=w490) -> ()  [unwired: 2 in, 9 out]
                }
              }
              frame True {
                n229 = Build Array(w499, w498) -> (w500:refnum<k7>[])
                n230 = for {
                  tunnel: w500 -> [w501] mode=indexing
                  w506 = sgl 0.5  # pfPitch
                  w503 = 1  # plDirSense
                  w507 = 1  # plUnits
                  n231 = invoke class="MG17Motor" method="SetStageAxisInfo"(reference=w501, "lChanID"=0 ("lLimitMode"), "fMinPos"=sgl 0.0, "fMaxPos"=sgl 4.0, "lUnits"=w507, "fPitch"=w506, "lDirSense"=w503) -> ()  [unwired: 2 in, 9 out]
                }
              }
            }
            n232 = property on="Go Home" class="Bool (strict)"("Val(Sgnl)"=FALSE ("Value (Signaling)")) -> ()  [unwired: 2 in, 2 out]
          }
          event "ExitSendCmd": Value Change {
            n233 = event-data() -> ()  [unwired: 1 in, 5 out]
          }
          event "Go Home": Value Change {
            n234 = event-data() -> ()  [unwired: 1 in, 5 out]
            n235 = Build Array(w513, w512) -> (w511:refnum<k7>[])
            n236 = for {
              tunnel: w511 -> [w516] mode=indexing
              tunnel: bool[] [FALSE, TRUE] -> [w517] mode=indexing
              tunnel: w509 -> [w515]
              n237 = invoke class="MG17Motor" method="SetAbsMovePos"(reference=w516, "lChanID"=w515, "fAbsPos"=sgl 2.0) -> (reference out=w520:refnum<k7>, error out=w518:errorcluster, "lChanID"=w519:i32)  [unwired: 2 in, 2 out]
              n238 = invoke class="MG17Motor" method="MoveAbsolute"(reference=w520, error in=w518, "lChanID"=w519, "bWait"=w517) -> ()  [unwired: 1 in, 5 out]
            }
            n239 = local write "Go Home"(FALSE ("Go Home")) -> ()
          }
          event "number of planes", "lines per plane", "Distance between\nscan lines (mm)", "Distance between\nplanes (mm)": Value Change {
            w523 = 4
            n240 = event-data() -> ()  [unwired: 1 in, 5 out]
            n241 = local read "Distance between\nscan lines (mm)"() -> (w534:sgl)
            n242 = local read "Distance between\nplanes (mm)"() -> (w535:sgl)
            n243 = local read "lines per plane"() -> (w528:u16)
            n244 = local read "number of planes"() -> (w529:u16)
            n245 = Decrement(x=w528) -> (x-1=w532:u16)
            n246 = Decrement(x=w529) -> (x-1=w533:u16)
            n247 = Multiply(x=w534, y=w532) -> (x*y=w530:sgl)
            n248 = Multiply(x=w535, y=w533) -> (x*y=w531:sgl)
            n249 = expression code="x/1000"(w531) -> (w527:sgl)
            "Cross Plane Length (mm)" <- w527
            n250 = expression code="x/1000"(w530) -> (w524:sgl)
            "Scan Plane Length (mm)" <- w524
            n251 = Greater?(x=w527, y=w523) -> (0:w526:bool)
            n252 = Greater?(x=w524, y=w523) -> (0:w522:bool)
            n253 = Or(x=w526, y=w522) -> (x .or. y?=w525:bool)
            n254 = case shown="True" w525 {
              frame False {
              }
              frame True {
                n255 = One Button Dialog(message="Total scan length cannot exceed 4 mm. Choose new values.") -> ()  [unwired: 1 in, 1 out]
              }
            }
          }
          event "Sample #": Value Change {
            # "Check if file name exists already."
            n256 = event-data() -> ("NewVal"=w541:u16)  [unwired: 1 in]
            n257 = local read "Root File Name"() -> (w542:string)
            n258 = call "File"("Beginning Text"=w542, "d"=w541) -> ("Result"=w539:string)  [unwired: 12 in, 1 out]
            n259 = Format Date/Time String(time format string (%c)="%Y-%m-%d") -> (date/time string=w543:string)  [unwired: 2 in]
            n260 = Build Path(base path="Save Folder", name or relative path=w543) -> (appended path=w540:path)
            n261 = Build Path(base path=w540, name or relative path=w539) -> (appended path=w538:path)
            n262 = call <vilib>:"Check if File or Folder Exists.vi"("path"=w538) -> ("file or folder exists?"=w537:bool)  [unwired: 8 in, 2 out]
            n263 = case shown="True" w537 {
              tunnel: w538 -> [_ w547]
              tunnel: w539 -> [_ w546]
              frame False {
              }
              frame True {
                n264 = Concatenate Strings(w546, "_Y*") -> (w551:string)
                n265 = List Folder(path=w547, pattern=w551) -> (filenames=w550:string[])  [unwired: 1 in, 4 out]
                n266 = Array Size(array=w550) -> (size(s)=w548:i32)
                n267 = case shown="1, Default" w548 {
                  frame 0 {
                  }
                  frame 1, Default {
                    n268 = One Button Dialog(message="File has been used already. Select a new file name.") -> ()  [unwired: 1 in, 1 out]
                  }
                }
              }
            }
          }
          event "Display as wavelength?": Value Change {
            n269 = event-data() -> ()  [unwired: 1 in, 5 out]
            n270 = case shown="True" "Display as wavelength?" {
              tunnel: u16 3712 -> [w557 w562]
              tunnel: [w556 w563] -> w554
              frame False {
                n271 = for {
                  N: w557 -> [_]
                  tunnel: [w558] -> w556 mode=indexing
                  i -> [w558]
                }
              }
              frame True {
                n272 = call "read_corr_coeff.vi"() -> ("A\n(Ax^2+Bx+C)"=w559:dbl, "B\n(Ax^2+Bx+C)"=w560:dbl, "C\n(Ax^2+Bx+C)"=w561:dbl)  [unwired: 1 in, 2 out]
                n273 = for {
                  N: w562 -> [_]
                  tunnel: w561 -> [w569]
                  tunnel: w560 -> [w568]
                  tunnel: w559 -> [w565]
                  tunnel: [w567] -> w563 mode=indexing
                  i -> [w566]
                  n274 = Multiply(x=w568, y=w566) -> (x*y=w570:dbl)
                  n275 = Compound Arithmetic op=MULTIPLY(w565, w566, w566) -> (w564:dbl)
                  n276 = Compound Arithmetic op=ADD(w569, w570, w564) -> (w567:dbl)
                }
              }
            }
            "X axis" <- w554
          }
        }
      }
    }
    frame #2 {
      n277 = case shown="2" w572 {
        tunnel: w574 -> [_ w581]
        tunnel: w573 -> [_ w580]
        frame 0, Default {
        }
        frame 2 {
          n278 = call <vilib>:"IMAQdx Stop Acquisition.vi"("error in"=w580, "Session In"=w581) -> ("error out"=w583:errorcluster, "Session Out"=w582:T4)  [unwired: 8 out]
          n279 = call <vilib>:"IMAQdx Unconfigure Acquisition.vi"("error in"=w583, "Session In"=w582) -> ("error out"=w578:errorcluster, "Session Out"=w579:T4)  [unwired: 8 out]
          n280 = call <vilib>:"IMAQdx Close Camera.vi"("error in"=w578, "Session In"=w579) -> ()  [unwired: 10 out]
        }
      }
      n281 = case shown="True" TRUE {
        tunnel: w576 -> [_ w585]
        tunnel: w575 -> [_ w584]
        frame False {
        }
        frame True {
          n282 = invoke class="MG17Motor" method="StopCtrl"(reference=w584) -> ()  [unwired: 2 in, 3 out]
          n283 = invoke class="MG17Motor" method="StopCtrl"(reference=w585) -> ()  [unwired: 2 in, 3 out]
        }
      }
      n284 = local write "ExitSendCmd"(FALSE ("ExitSendCmd")) -> ()
    }
  }
